vi "Write to XML File(string).vi"(6 "Standalone? (T)":bool=TRUE, 8 "error in (no error)":errorcluster, 9 "XML Encoding":string, 10 "XML Input":string, 11 "XML File Path":path) -> (0 "error out":errorcluster, 2 "XML String":string, 3 "XML File Path(duplicate)":path)   [LabVIEW 2012]
doc: "Writes a text string of XML data with accompanying header tags to a text file. Wire data to the <B>XML Input</B> input to determine the polymorphic instance to use or manually select the instance. All XML data must follow the standard LabVIEW XML schema."
panel:
  in  "Prompt":string="Select Path to XML File"
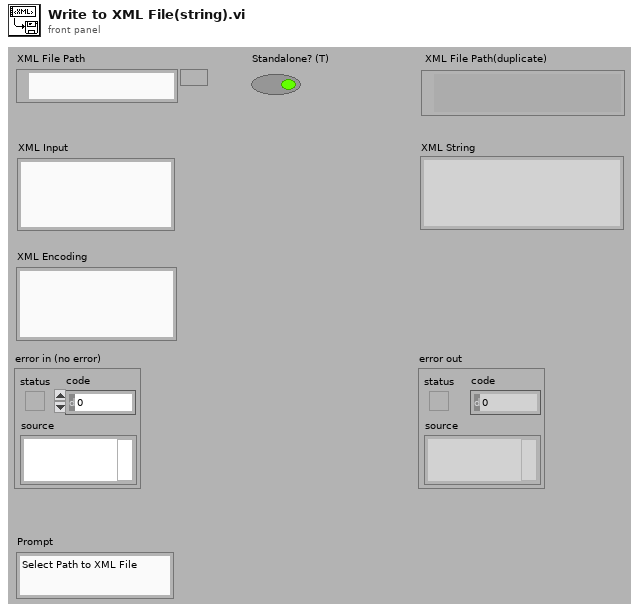
[diagram p1: front panel]
types:
  T1 = enum16{"open", "open or create", "create or replace", "create", "open (read only)"}
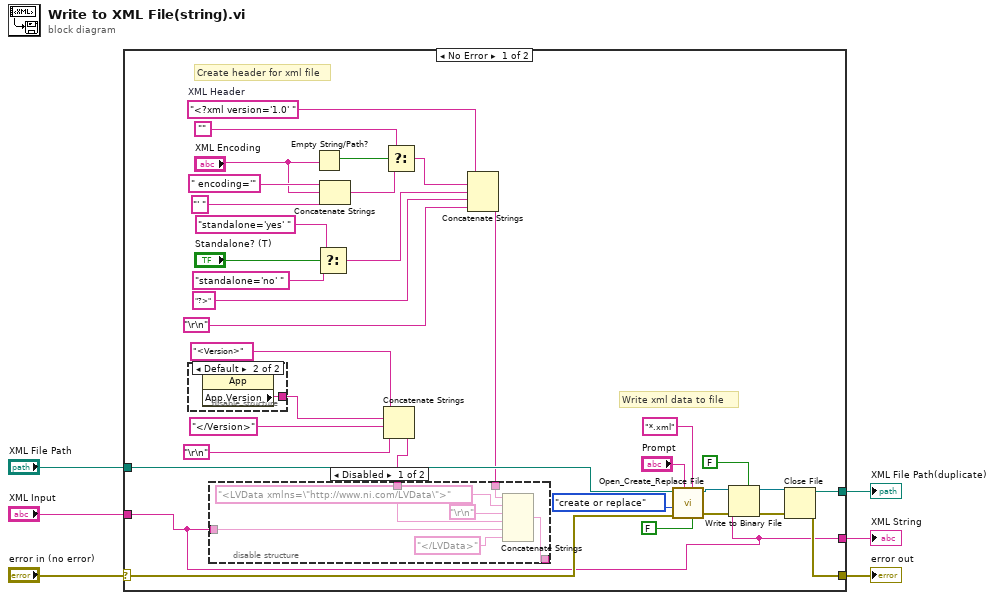
[diagram p0: block diagram]
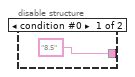
[diagram p3: hidden frame]
diagram:
  n1 = case shown="No Error" "error in (no error)" {
    selector: "error in (no error)" -> [w16 w52]
    tunnel: [w17 w52] -> w5
    tunnel: "XML Input" -> [w7 w51]
    tunnel: [w7 w51] -> w3
    tunnel: [w12 w50] -> w2
    tunnel: "XML File Path" -> [w21 w50]
    frame No Error {
      w40 = "<?xml version='1.0' "  # XML Header
      # "Create header for xml file"
      # "Write xml data to file"
      n2 = disable-structure shown="Default" {
        disable-tunnel: ["8.5" ("App.Version") w49] -> w25
        frame condition #0 {
        }
        frame condition #1 (active) {
          n3 = property class="App"() -> ("App.Version"=w49:string)  [unwired: 2 in, 2 out]
        }
      }
      n4 = Empty String/Path?(string/path="XML Encoding") -> (empty?=w33:bool)
      n5 = Select(t="standalone='yes' " ("Substring"), s="Standalone? (T)", f="standalone='no' " ("Substring")) -> (s? t:f=w27:string)
      n6 = Concatenate Strings(" encoding='", "XML Encoding", "' " ("Substring")) -> (w32:string)
      n7 = Concatenate Strings("<Version>", w25, "</Version>", "\r\n") -> (w22:string)
      n8 = Select(t="", s=w33, f=w32) -> (s? t:f=w30:string)
      n9 = Concatenate Strings(w40, w30, w27, "?>" ("Substring"), "\r\n") -> (w8:string)
      n10 = disable-structure shown="Disabled" {
        disable-tunnel: w22 -> [w47 _]
        disable-tunnel: w8 -> [w46 _]
        disable-tunnel: w7 -> [w45 _]
        disable-tunnel: [w41 _] -> _
        frame Disabled {
          n11 = Concatenate Strings(w46, "<LVData xmlns=\"http://www.ni.com/LVData\">" ("Substring"), "\r\n", w47, w45, "</LVData>" ("Substring")) -> (w41:string)
        }
        frame Enabled {
        }
      }
      n12 = call <vilib>:"Open_Create_Replace File.vi"("advisory dialog? (display:T)"=FALSE, "pattern"="*.xml", "prompt"="Prompt", "error in (no error)"=w16, "function (open:0)"=T1."create or replace", "file path"=w21) -> ("error out"=w19:errorcluster, "refnum"=w15:refnum<file>)  [unwired: 2 in, 2 out]
      n13 = Write to Binary File(file (use dialog)=w15, data=w7, error in=w19, 5:FALSE ("prepend array or string size? (T)")) -> (refnum out=w13:refnum<file>, error out=w18:errorcluster)  [unwired: 3 out]
      n14 = Close File(refnum=w13, error in=w18) -> (path=w12:path, error out=w17:errorcluster)
    }
    frame Error {
    }
  }
  "error out" <- w5
  "XML String" <- w3
  "XML File Path(duplicate)" <- w2
